vi "Digital Out Write.vi"(8 "error in (no error)":errorcluster, 10 "Port Mask":u64, 11 "MSX-E3701 in":refnum<class "MSX-E3701.lvclass">) -> (0 "error out":errorcluster, 3 "MSX-E3701 out":refnum<class "MSX-E3701.lvclass">)   [LabVIEW 2014, in "MSX-E3701.lvlib" / "MSX-E3701.lvclass"]
doc: "Escribe el puerto de salida para setear las DIO."
uses:
  MSX-E3701.lvclass
  MSX-E3701.lvclass/MSX-E3701.ctl
  API/MSX-E3701_dll.lvlib
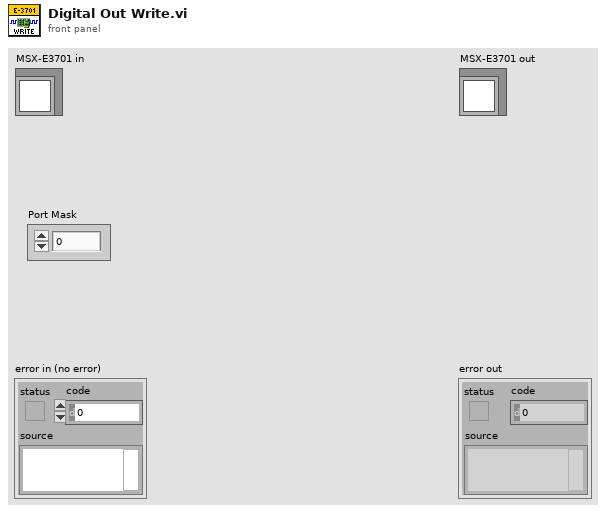
[diagram p1: front panel]
types:
  T1 = typedef "MSX-E3701_dll.lvlib/Connection Data.ctl" = cluster{"MX370x refnum":refnum<k24>, "IP":string, "Connection ID ":refnum<k5>, "MXCommon refnum":refnum<k24>}
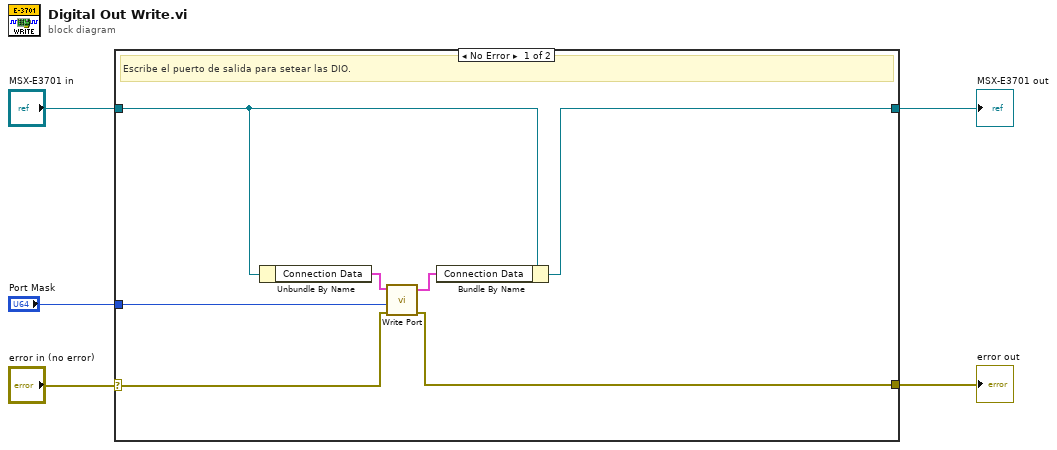
[diagram p0: block diagram]
diagram:
  n1 = case shown="No Error" "error in (no error)" {
    selector: "error in (no error)" -> [w9 w14]
    tunnel: [w10 w14] -> w4
    tunnel: [w6 w13] -> w2
    tunnel: "MSX-E3701 in" -> [w7 w13]
    tunnel: "Port Mask" -> [w8 _]
    frame No Error {
      # "Escribe el puerto de salida para setear las DIO."
      n2 = Unbundle By Name(w7) -> ("Connection Data"=w12:T1)
      n3 = call "Write Port.vi"("error in (no error)"=w9, "Port Mask"=w8, "Connection Data In"=w12) -> ("error out"=w10:errorcluster, "Connection Data Out"=w11:T1)  [unwired: 7 in]
      n4 = Bundle By Name(cluster=w7, "Connection Data"=w11) -> (w6:refnum<class "MSX-E3701.lvclass">)
    }
    frame Error {
    }
  }
  "error out" <- w4
  "MSX-E3701 out" <- w2
